vi "DB Read IOlist.vi"() -> (1 "output cluster":T1)   [LabVIEW 2015]
uses:
  <vilib>/Utility/file.llb/Read Delimited Spreadsheet (string).vi
panel:
  out "Application Directory":path
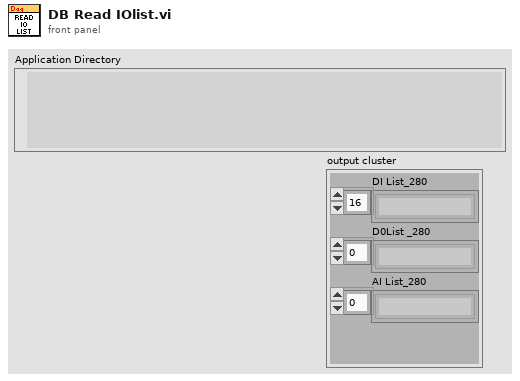
[diagram p1: front panel]
types:
  T1 = cluster{"DI List_280":string[], "D0List _280":string[], "AI List_280":string[]}
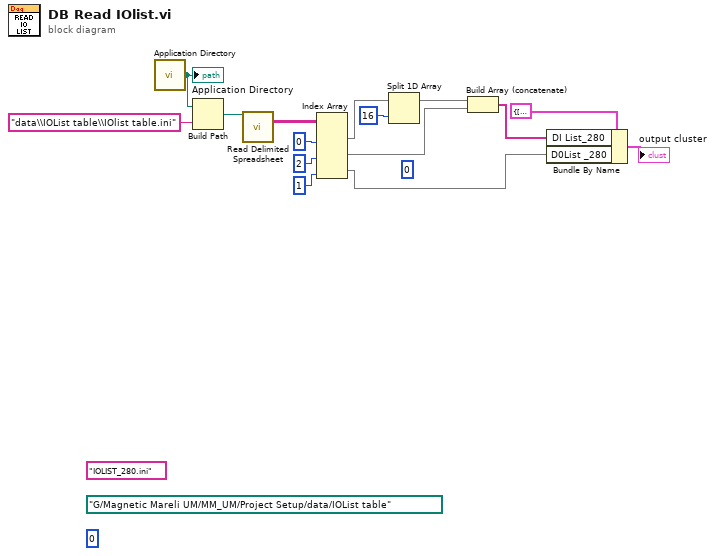
[diagram p0: block diagram]
diagram:
  (unwired) "IOLIST_280.ini"
  (unwired) 0 ("index")
  (unwired) path "G:/Magnetic Mareli UM/MM_UM/Project Setup/data/IOList table" ("base path")
  (unwired) 0 ("index (page)")
  n1 = call <vilib>:"Application Directory.vi"() -> ("Application Directory"=w6:path)
  "Application Directory" <- w6
  n2 = Build Path(base path=w6, name or relative path="data\\IOList table\\IOlist table.ini") -> (appended path=w2:path)
  n3 = call-poly <vilib>:"Read Delimited Spreadsheet.vi"("file path (dialog if empty)"=w2) -> ("all rows"=w3:string[][])  [unwired: 9 in, 5 out]
  n4 = Index Array(array=w3, index (col) #1=0 ("disabled index (col)"), index (col) #2=2 ("disabled index (col)"), index (col) #3=1 ("disabled index (col)")) -> (element #1=w9:string[], element #2=w1:string[], element #3=w15:string[])  [unwired: 3 in]
  n5 = Split 1D Array(array=w9, index=16) -> (first subarray=w11:string[])  [unwired: 1 out]
  n6 = Build Array (concatenate)(w11, w1) -> (w14:string[])
  n7 = Bundle By Name(cluster=T1 {"DI List_280"=[" Start PB (P0.0) ", "Emergency Stop (P0.1)", "Reset PB (P0.2)", "Home PB (P0.3)", "Main Pressure Signal (P0.4)", "Safety Signal-1 (P0.5)", "Safety Signal-2 (P0.6)", "Fixture Sliding Servo Home RS (P0.7)", "Fixture Sliding Servo Fault Signal (P0.8)", "LCD pressing Servo Home RS (P0.9)", "LCD pressing Servo fault Signal (P0.10)", "Spare", "Spare", "Spare", "Spare", "Model conformation PX-1 (AI2)", "Model conformation PX-2 (AI3)", "Diffuser height checking Sensor-1 (AI4)", "Diffuser height checking Sensor-2 (AI5)", "Panel Door Open Signal (AI6)", "Component CNF Sensor on Ionizer (AI7)", "Bi-adhesive tube Waste Collection bin CNF Sensor (AI8)", "Photo Prism presence Sensor (AI9)", "Lightbox presence CNF Sensor (AI10)", "Diffuser presence CNF Sensor (AI11)", "Photo prism height checking UP CYL Rs (AI12)", "Photo prism height checking DWN CYL  Rs (AI13)", "Camera slide Cyl Fwd Rs (AI14)", "Camera slide Cyl Rev Rs (AI15)", "LCD Display Rotating Unit Actuator Cyl CW PX (AI16)", "LCD Display Rotating Unit Actuator Cyl CCW PX (AI17)", "Fixture clamping Cyl Fwd Rs (AI18)", "Fixture clamping Cyl Rev Rs (AI19)", "Clip pulling unit Cyl Fwd Rs (AI20)", "Clip pulling unit Cyl Rev Rs (AI21)", "Clip clamp unit Cyl Fwd Rs (A22)", "Clip clamp unit Cyl Rev Rs (AI23)", "Barcode Scanner Ready Signal (AI24)", "Spare", "Spare", "Spare", "Spare", "Spare", "Spare", "Spare"], "D0List _280"=["Ionizer ON Sol (P0.16)", "Fixture Slide Servo Fault Reset (P0.17)", "LCD pressing servo Fault Reset (P0.18)", "Fixture Slide servo Brake ON Cmd (P0.19)", "Fixture Slide Servo Direction Command (P0.20)", "LCD pressing Servo Direction Command (P0.21)", "LCD pressing Servo Brake ON Cmd (P0.22)", "Photo prism height checking UP CYL Sol (P0.23)", "Photo prism height checking DWN CYL  Sol (P0.24)", "Camera slide Cyl Fwd Sol (P0.25)", "Camera slide Cyl Rev Sol (P0.26)", "LCD Display Rotating Unit Actuator Cyl CW Sol (P0.27)", "LCD Display Rotating Unit Actuator Cyl CCW Sol (P0.28)", "Fixture clamping Cyl Fwd Sol (P0.29)", "Fixture clamping Cyl Rev Sol (P0.30)", "Clip pulling unit Cyl Fwd Sol (P0.31)", "Clip pulling unit Cyl Rev Sol (P1.0)", "Clip clamp unit Cyl Up Sol (P1.1)", "Clip clamp unit Cyl Dwn Sol (P1.2)", "Optional required based Barcode Trigger Cmd (P1.3)", "TWL Red /Fault with Buzzer (P1.4)", "TWL Green/OK (P1.5)", "TWL Yellow/ Running (P1.6)", "Spare", "Spare", "Spare", "Spare", "Spare", "Fixture Slide Servo Pulse Command (P2.4)", "LCD pressing Servo Pulse Command (P2.5)", "Spare", "Spare"], "AI List_280"=[]} ("Cluster 2"), "DI List_280"=w14, "D0List _280"=w15) -> (→"output cluster":T1)
